vi "get-cam-names.vi"(8 "error in (no error)":errorcluster) -> (0 "error out":errorcluster, 3 "cam names":string[](array[string]))   [LabVIEW 2024]
uses:
  <vilib>/vision/driver/NI_Vision_Acquisition_Software.lvlib
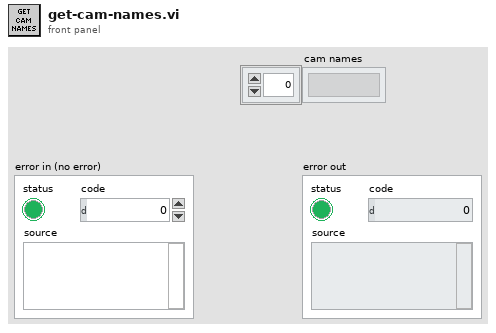
[diagram p1: front panel]
types:
  T1 = cluster{"Type":u32, "Version":u32, "Flags":u32, "SerialNumberHigh":u32, "SerialNumberLow":u32, "BusType":u32, "InterfaceName":string, "VendorName":string, "ModelName":string, "CameraFileName":string, "CameraAttributeURL":string}[]
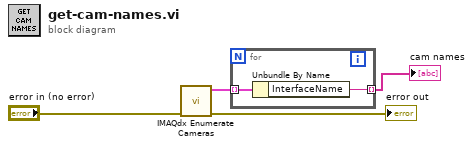
[diagram p0: block diagram]
diagram:
  n1 = call <vilib>:"IMAQdx Enumerate Cameras.vi"("error in"="error in (no error)") -> ("error out"=→"error out":errorcluster, "Camera Information Array"=w3:T1)  [unwired: 9 in]
  n2 = for {
    tunnel: w3 -> [w6] mode=indexing
    tunnel: [w5] -> w1 mode=indexing
    n3 = Unbundle By Name(w6) -> ("InterfaceName"=w5:string)
  }
  "cam names" <- w1
